vi "Map to JSON.vi"(4 "LVClass Serializer":refnum<class "JSONtext LVClass Serializer.lvclass">, 5 "enable LabVIEW extensions?":bool, 6 "Pretty Print?":bool, 8 "error in (no error)":errorcluster, 11 "Map":variant) -> (0 "error out":errorcluster, 2 "<JSON>":string)   [LabVIEW 2020, in "JSONtext.lvlib" / "SetMap.lvlib"]
uses:
  <vilib>/JDP Science/JSONtext/support/Set Map/SetMap.lvlib
  <vilib>/JDP Science/JSONtext/LVClass Serializer/JSONtext LVClass Serializer.lvclass
  <vilib>/JDP Science/JSONtext/support/Set Map/SubType.vi
  <vilib>/JDP Science/JSONtext/support/Format JSON Array Text.vi
  <vilib>/JDP Science/JDP Science Common Utilities/JDP Utility.lvlib
  <vilib>/JDP Science/JSONtext/JSONtext.lvlib
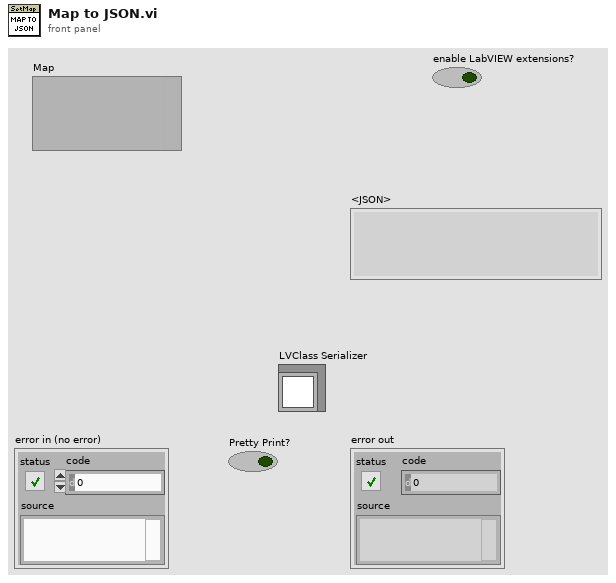
[diagram p1: front panel]
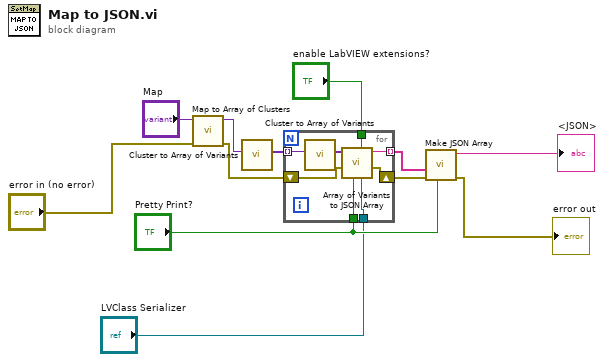
[diagram p0: block diagram]
diagram:
  n1 = call <vilib>:"Map to Array of Clusters.vi"("error in"="error in (no error)", "Map"="Map") -> ("error out"=w10:errorcluster, "Array of Clusters (key-value)"=w2:variant)  [unwired: 8 in]
  n2 = call <vilib>:"Cluster to Array of Variants.vi"("Cluster"=w2) -> ("Array of Cluster Elements"=w3:variant[])  [unwired: 10 in]
  n3 = for {
    tunnel: w3 -> [w20] mode=indexing
    tunnel: [w18] -> w4 mode=indexing
    tunnel: "Pretty Print?" -> [w17]
    tunnel: "enable LabVIEW extensions?" -> [w16]
    shift-right: [w14] -> w11
    shift-left: w10 -> [w15]
    tunnel: "LVClass Serializer" -> [w13]
    n4 = call <vilib>:"Cluster to Array of Variants.vi"("Cluster"=w20) -> ("Array of Cluster Elements"=w19:variant[])  [unwired: 10 in]
    n5 = call <vilib>:"Array of Variants to JSON Array.vi"("LVClass Serializer"=w13, "enable LabVIEW extensions? (T)"=w16, "Pretty Print?"=w17, "error in (no error)"=w15, "Array of Variants"=w19) -> ("error out"=w14:errorcluster, "<JSON>"=w18:string)  [unwired: 5 in]
  }
  n6 = call <vilib>:"Make JSON Array.vi"("Pretty Print?"="Pretty Print?", "error in (no error)"=w11, "JSON Elements"=w4) -> ("error out"=→"error out":errorcluster, "<JSON>"=→"<JSON>":string)  [unwired: 7 in]
